vi "_DebugV1.0+no344.vi"() -> ()   [LabVIEW 2017]
uses:
  <vilib>/Instr/_visa.llb/VISA Configure Serial Port (Instr).vi
panel:
  out "Vdac/Vch1":cluster{dbl[], dbl[]}(graph)
  out "Numeric":i32
  out "Vdac/Vout":cluster{dbl[], dbl[]}(graph)
  out "344":cluster{dbl[], dbl[]}(graph)
  out "DAC1":cluster{dbl[], dbl[]}(graph)
  out "DAC1volt, V":dbl
  out "Bytes at Port":u32
  out "RecTry":i32
  out "OutVoltage, V":dbl
  out "Knob":u32
  out "Current, mA":dbl format="%#_4g"
  out "Channel 1, V":dbl format="%#_5g"
  in  "Stop Button":bool
  in  "Start Button":bool
  out "VoltageArray, V":dbl[](array[numeric])
  in  "Step, V":dbl
  in  "Amplitude, V":dbl
  in  "LOG file":path
  in  "COM port":refnum<visa-resource-name>
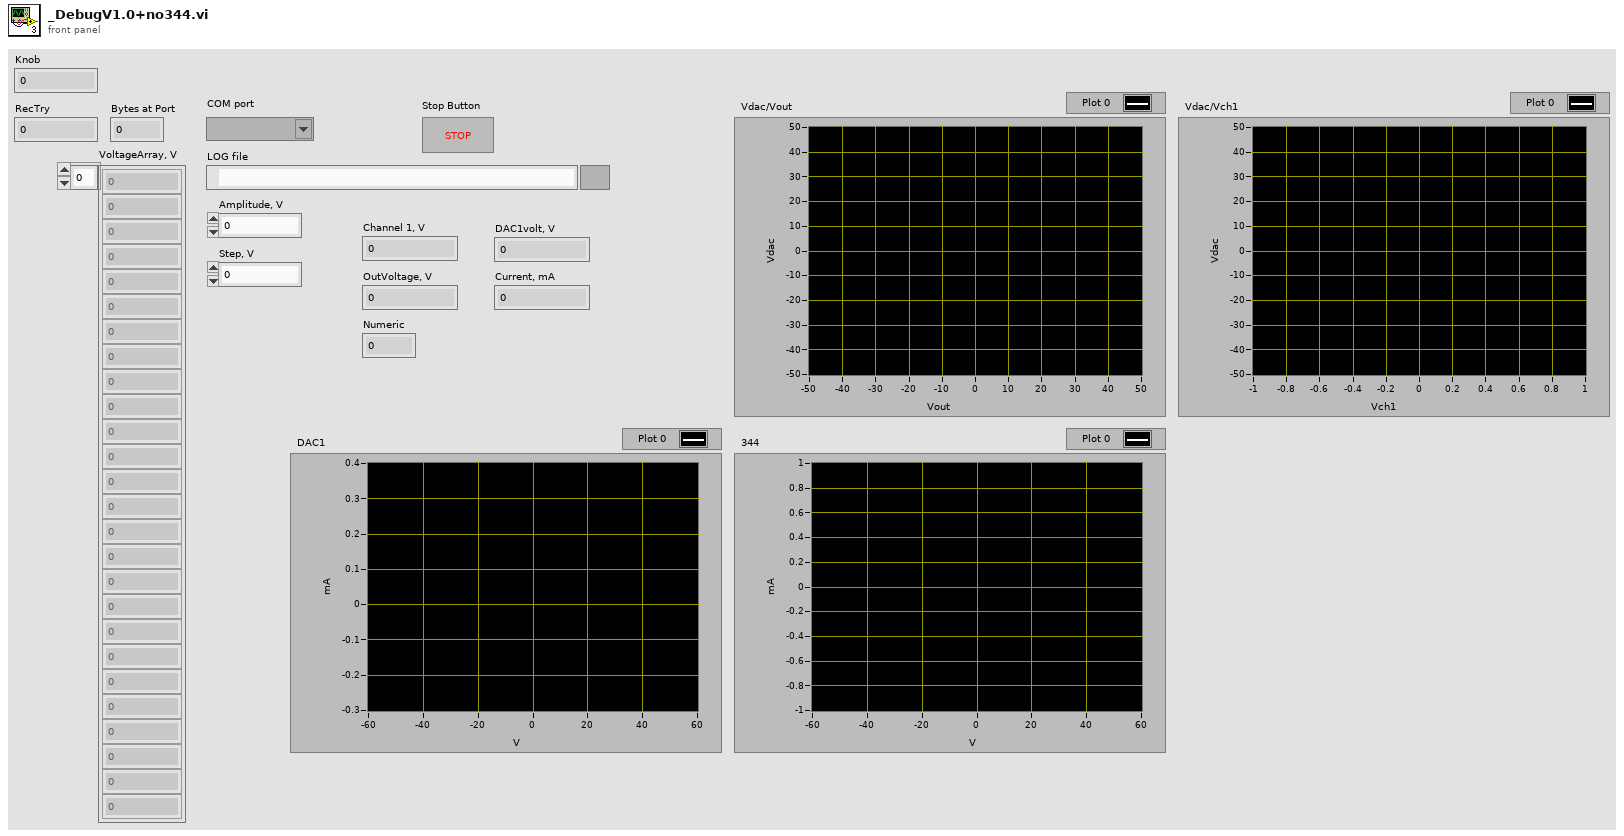
[diagram p1: front panel]
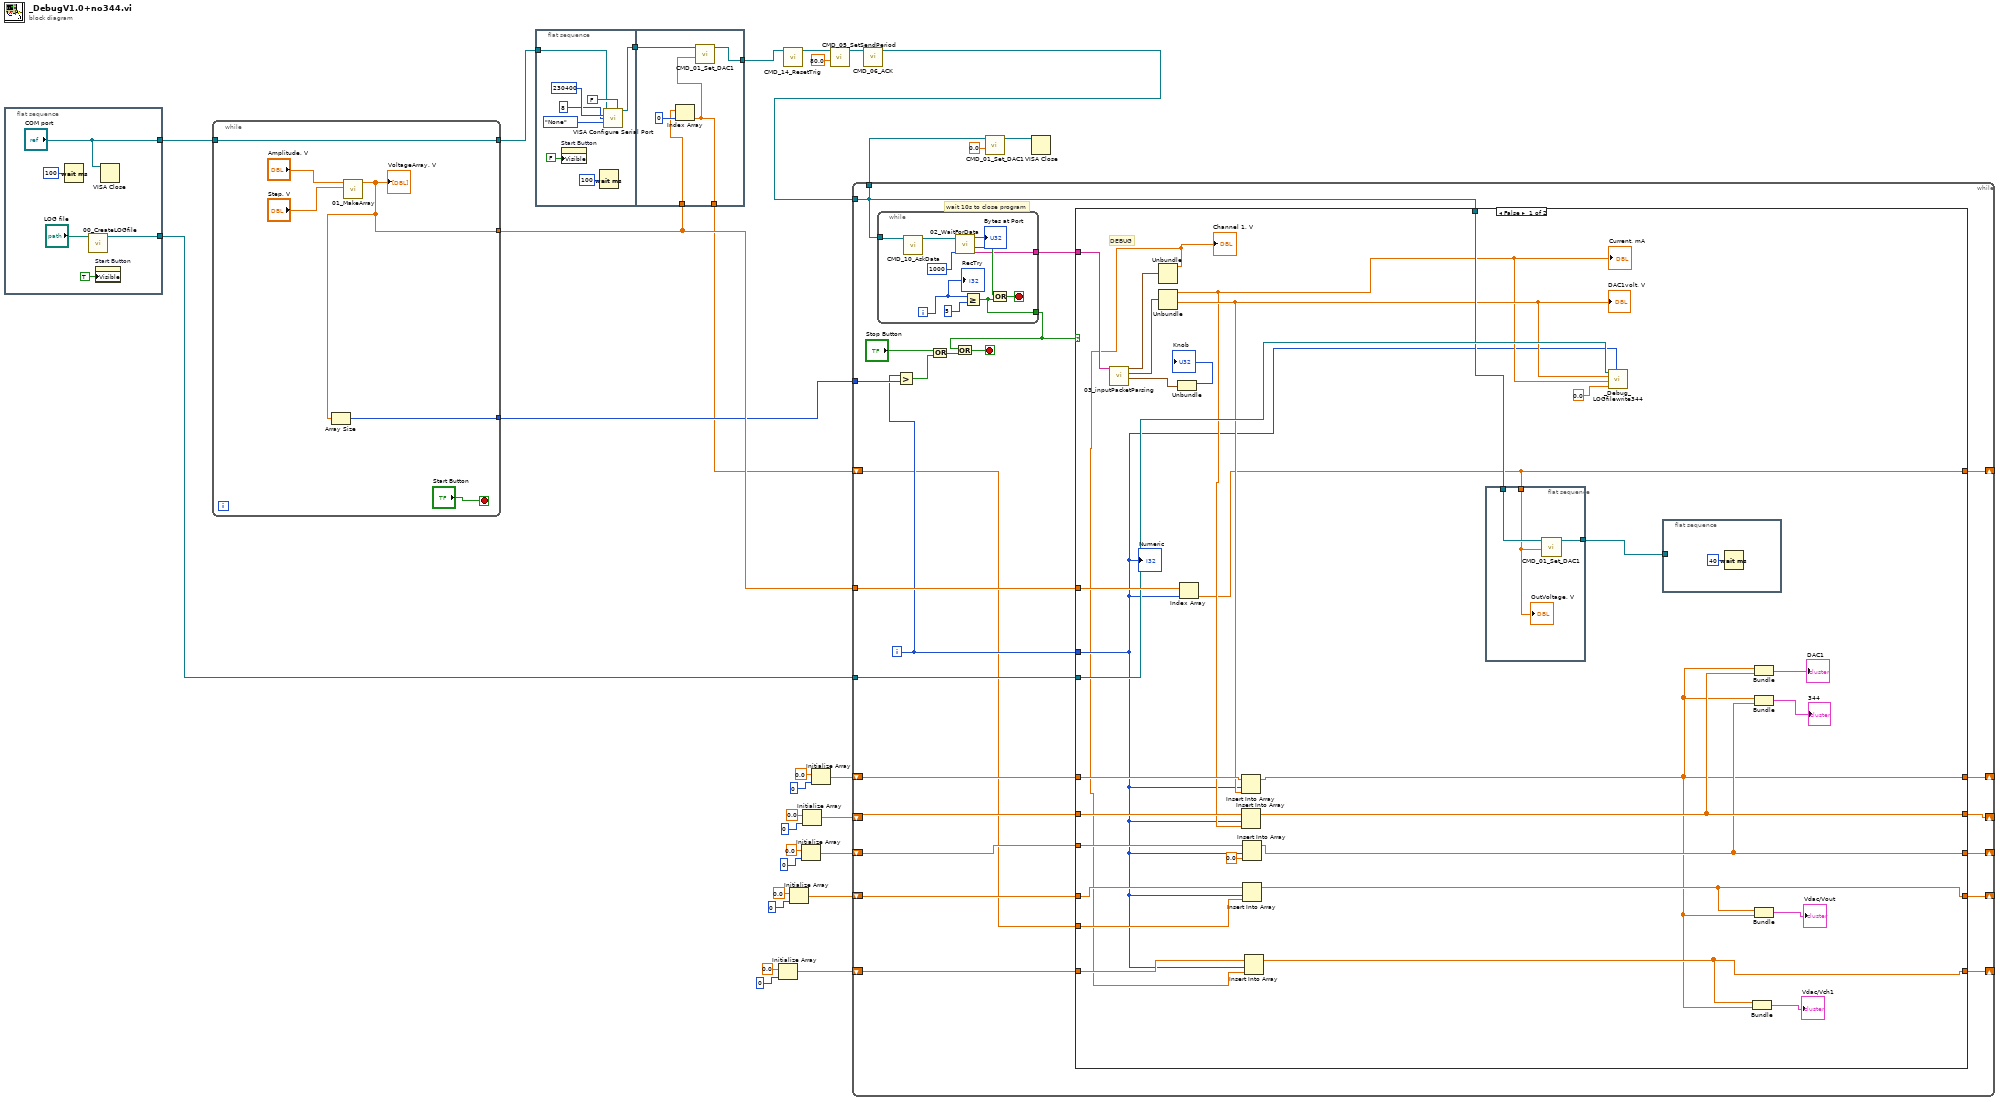
[diagram p0: block diagram]
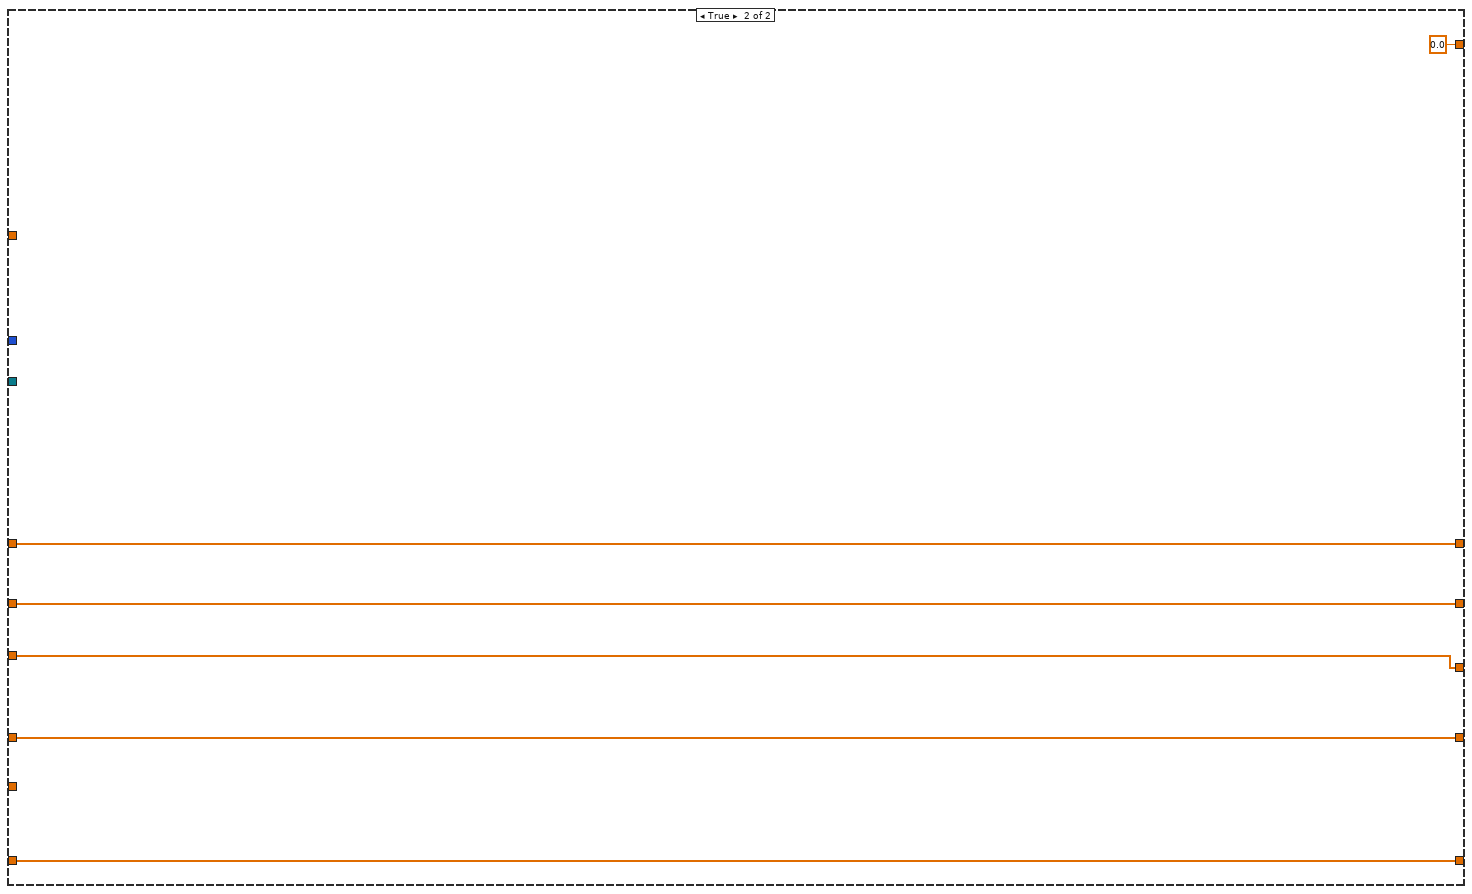
[diagram p2: hidden frame]
diagram:
  n1 = flat-sequence {
    tunnel: ["COM port"] -> w30
    tunnel: [w32] -> w28
    frame #0 {
      n2 = Wait (ms)(milliseconds to wait=u32 100) -> ()  [unwired: 1 out]
      n3 = call "00_CreateLOGfile.vi"("LOG file"="LOG file") -> ("refnum out"=w32:refnum<file>)  [unwired: 10 in]
      n4 = property on="Start Button" class="Bool"("Visible"=TRUE) -> ()  [unwired: 2 in, 2 out]
      n5 = VISA Close(VISA resource name="COM port") -> ()  [unwired: 1 in, 1 out]
    }
  }
  n6 = while {
    tunnel: w30 -> [w38]
    tunnel: [w38] -> w29
    tunnel: [w37] -> w18
    tunnel: [w36] -> w17
    stop <- "Start Button" stop-if-true
    n7 = call "01_MakeArray.vi"("Amp"="Amplitude, V", "Step"="Step, V") -> ("Array"=w37:dbl[])  [unwired: 8 in]
    "VoltageArray, V" <- w37
    n8 = Array Size(array=w37) -> (size(s)=w36:i32)
  }
  n9 = flat-sequence {
    tunnel: w29 -> [w45]
    tunnel: [w44] -> w19
    tunnel: [w53] -> w26
    tunnel: w19 -> [w52]
    tunnel: w18 -> [w51]
    tunnel: [w50] -> w4
    frame #0 {
      n10 = property on="Start Button" class="Bool"("Visible"=FALSE) -> ()  [unwired: 2 in, 2 out]
      n11 = Wait (ms)(milliseconds to wait=u32 100) -> ()  [unwired: 1 out]
      n12 = call-poly "VISA Configure Serial Port"("VISA resource name"=w45, "Enable Termination\nChar (T)"=FALSE ("Enable Termination\nChar (T)"), "baud rate (9600)"=u32 230400, "data bits (8)"=u16 8, "parity (0:none)"=enum16{"None", "Odd", "Even", "Mark", "Space"}."None") -> ("VISA resource name out"=w44:refnum<visa-resource-name>)  [unwired: 9 in, 1 out]
    }
    frame #1 {
      n13 = Index Array(array=w51, index=0) -> (element=w50:dbl)
      n14 = call "CMD_01_Set_DAC1.vi"("Input, V"=w50, "VISA resource name"=w52) -> ("VISA resource name out"=w53:refnum<visa-resource-name>)  [unwired: 9 in]
    }
  }
  n15 = Initialize Array(0.0 ("element"), 0 ("dimension size")) -> (w1:dbl[])
  n16 = call "CMD_14_ResetTrig.vi"("VISA resource name"=w26) -> ("VISA resource name out"=w22:refnum<visa-resource-name>)  [unwired: 10 in]
  n17 = Initialize Array(0.0 ("element"), 0 ("dimension size")) -> (w5:dbl[])
  n18 = Initialize Array(0.0 ("element"), 0 ("dimension size")) -> (w8:dbl[])
  n19 = Initialize Array(0.0 ("element"), 0 ("dimension size")) -> (w11:dbl[])
  n20 = Initialize Array(0.0 ("element"), 0 ("dimension size")) -> (w16:dbl[])
  n21 = call "CMD_05_SetSendPeriod.vi"("Period, ms"=80.0, "VISA resource name"=w22) -> ("VISA resource name out"=w21:refnum<visa-resource-name>)  [unwired: 9 in]
  n22 = call "CMD_06_ACK.vi"("VISA resource name"=w21) -> ("VISA resource name out"=w20:refnum<visa-resource-name>)  [unwired: 10 in]
  n23 = while {
    tunnel: w20 -> [w72]
    tunnel: [w72] -> w27
    tunnel: w18 -> [w73]
    tunnel: w28 -> [w74]
    tunnel: w17 -> [w69]
    shift-right: [w63] -> _
    shift-left: w16 -> [w64]
    shift-right: [w62] -> _
    shift-left: w11 -> [w65]
    shift-right: [w61] -> _
    shift-left: w8 -> [w66]
    shift-right: [w59] -> _
    shift-left: w5 -> [w60]
    shift-right: [w58] -> _
    shift-left: w4 -> [w57]
    shift-right: [w55] -> _
    shift-left: w1 -> [w56]
    i -> [w67]
    stop <- w77 stop-if-true
    # "wait 10s to close program"
    n24 = while {
      tunnel: w72 -> [w120]
      tunnel: [w123] -> w76
      tunnel: [w124] -> w75
      i -> [w122]
      stop <- w126 stop-if-true
      n25 = call "CMD_10_AskData.vi"("VISA resource name"=w120) -> ("VISA resource name out"=w119:refnum<visa-resource-name>)  [unwired: 10 in]
      n26 = call "02_WaitForData.vi"("WaitTimeoutMS"=u32 1000, "VISA"=w119) -> ("Buffer"=w124:string, "Bytes at Port"=→"Bytes at Port":u32, "Data Recived"=w125:bool)  [unwired: 7 in]
      n27 = Greater Or Equal?(x=w122, y=5) -> (x >= y?=w123:bool)
      n28 = Or(x=w125, y=w123) -> (x .or. y?=w126:bool)
      "RecTry" <- w122
    }
    n29 = Greater?(x=w67, y=w69) -> (0:w68:bool)
    n30 = Or(x="Stop Button", y=w68) -> (x .or. y?=w71:bool)
    n31 = Or(x=w76, y=w71) -> (x .or. y?=w77:bool)
    n32 = case shown="False" w76 {
      tunnel: w75 -> [w102 _]
      tunnel: w74 -> [w103 _]
      tunnel: w67 -> [w85 _]
      tunnel: w73 -> [w104 _]
      tunnel: w72 -> [w101 _]
      tunnel: w66 -> [w100 w116]
      tunnel: w65 -> [w99 w117]
      tunnel: w64 -> [w98 w118]
      tunnel: [w80 w118] -> w63
      tunnel: [w95 w117] -> w62
      tunnel: [w94 w116] -> w61
      tunnel: w60 -> [w91 w115]
      tunnel: [w82 w115] -> w59
      tunnel: [w90 0.0] -> w58
      tunnel: w57 -> [w89 _]
      tunnel: w56 -> [w86 w113]
      tunnel: [w81 w113] -> w55
      frame False {
        # "DEBUG"
        n33 = call "03_inputPacketParsing.vi"("string"=w102) -> ("Service state"=w105:cluster{u8, u8}, "DAC state"=w108:cluster{dbl, dbl, dbl, dbl}, "Voltage"=w106:cluster{dbl, dbl, dbl, dbl})  [unwired: 6 in, 2 out]
        n34 = Unbundle(w106) -> (w84:dbl)  [unwired: 3 out]
        "Channel 1, V" <- w84
        n35 = Unbundle(w108) -> (w96:dbl, w97:dbl)  [unwired: 2 out]
        "Current, mA" <- w96
        "DAC1volt, V" <- w97
        n36 = Unbundle(w105) -> (→"Knob":u8)  [unwired: 1 out]
        n37 = Index Array(array=w104, index=w85) -> (element=w90:dbl)
        n38 = Insert Into Array(array=w98, index=w85, new element=w97) -> (w80:dbl[])
        n39 = Insert Into Array(array=w99, index=w85, new element=w96) -> (w95:dbl[])
        n40 = Insert Into Array(array=w100, index=w85, new element=0.0 ("new element/subarray")) -> (w94:dbl[])
        n41 = Insert Into Array(array=w91, index=w85, new element=w89) -> (w82:dbl[])
        n42 = Insert Into Array(array=w86, index=w85, new element=w84) -> (w81:dbl[])
        n43 = flat-sequence {
          tunnel: w90 -> [w110]
          tunnel: w101 -> [w112]
          tunnel: [w111] -> w87
          frame #0 {
            n44 = call "CMD_01_Set_DAC1.vi"("Input, V"=w110, "VISA resource name"=w112) -> ("VISA resource name out"=w111:refnum<visa-resource-name>)  [unwired: 9 in]
            "OutVoltage, V" <- w110
          }
        }
        n45 = call "_Debug_LOGfilewrite344.vi"("N"=w85, "344cur"=0.0, "DAC1cur"=w96, "DAC1volt2"=w97, "refnum out"=w103) -> ()  [unwired: 7 in]
        n46 = flat-sequence {
          tunnel: w87 -> [_]
          frame #0 {
            n47 = Wait (ms)(milliseconds to wait=u32 40) -> ()  [unwired: 1 out]
          }
        }
        n48 = Bundle(w81, w80) -> (→"Vdac/Vch1":cluster{dbl[], dbl[]})  [unwired: 1 in]
        n49 = Bundle(w80, w95) -> (→"DAC1":cluster{dbl[], dbl[]})  [unwired: 1 in]
        n50 = Bundle(w80, w94) -> (→"344":cluster{dbl[], dbl[]})  [unwired: 1 in]
        n51 = Bundle(w82, w80) -> (→"Vdac/Vout":cluster{dbl[], dbl[]})  [unwired: 1 in]
        "Numeric" <- w85
      }
      frame True {
      }
    }
  }
  n52 = call "CMD_01_Set_DAC1.vi"("Input, V"=0.0, "VISA resource name"=w27) -> ("VISA resource name out"=w24:refnum<visa-resource-name>)  [unwired: 9 in]
  n53 = VISA Close(VISA resource name=w24) -> ()  [unwired: 1 in, 1 out]
